vi "ControlEnhanced - BackupCopy.vi"() -> ()   [LabVIEW 2018]
uses:
  <vilib>/Platform/TimedLoop/XDataNode/timing_clust.ctl
  <vilib>/Platform/TimedLoop/XDataNode/nitl_modes.ctl
  <vilib>/Platform/TimedLoop/XDataNode/wakeup.ctl
  <vilib>/myRIO/Instrument Drivers/Onboard IO/AI/typedefs/AI Reference.ctl
  <vilib>/myRIO/Common/Instrument Driver Framework/Utilities/typedefs/myRIO Generic Hardware Reference.ctl
  <vilib>/myRIO/Common/Instrument Driver Framework/Utilities/typedefs/Hardware Version Enum.ctl
  <vilib>/myRIO/Common/Instrument Driver Framework/Utilities/typedefs/myRIO v1.0 Reference.ctl
  <vilib>/myRIO/Common/Instrument Driver Framework/Utilities/typedefs/Generic FPGA Reference.ctl
  <vilib>/myRIO/Common/Instrument Driver Framework/myRIO v1.0/AI/typedefs/AI Channels List.ctl
  <vilib>/myRIO/Common/Instrument Driver Framework/myRIO v1.0/AI/typedefs/AI Channels Enum.ctl
  <vilib>/myRIO/Common/Instrument Driver Framework/Utilities/typedefs/Analog Scaling Constants List.ctl
  <vilib>/myRIO/Common/Instrument Driver Framework/Utilities/typedefs/Analog Scaling Constants.ctl
  <vilib>/userdefined/High Color/nirio_resource_hc.ctl
  <vilib>/myRIO/Instrument Drivers/Onboard IO/AO/typedefs/AO Reference.ctl
  <vilib>/myRIO/Common/Instrument Driver Framework/myRIO v1.0/AO/typedefs/AO Channels List.ctl
  <vilib>/myRIO/Common/Instrument Driver Framework/myRIO v1.0/AO/typedefs/AO Channels Enum.ctl
  <vilib>/myRIO/Common/Instrument Driver Framework/Utilities/vis/Is FPGA Ref Available.vi
  <vilib>/myRIO/Common/Instrument Driver Framework/myRIO v1.0/AI/vis/myRIO v1.1 Open AI.vi
  <vilib>/myRIO/Instrument Drivers/Onboard IO/AI/vis/Read.vi
  <vilib>/myRIO/Common/Instrument Driver Framework/myRIO v1.0/AO/vis/myRIO v1.1 Open AO.vi
  <vilib>/myRIO/Instrument Drivers/Onboard IO/AO/vis/Write.vi
  <vilib>/myRIO/Common/Instrument Driver Framework/Utilities/vis/Validate Channels.vi
  <vilib>/myRIO/Common/Instrument Driver Framework/myRIO v1.0/AI/vis/myRIO v1.0 Reserve AI.vi
  <vilib>/myRIO/Common/Instrument Driver Framework/myRIO v1.0/AO/vis/myRIO v1.0 Reserve AO.vi
  <vilib>/myRIO/Common/Instrument Driver Framework/myRIO v1.0/AI/vis/myRIO v1.0 Build MUX Configuration AI.vi
  <vilib>/myRIO/Common/Instrument Driver Framework/myRIO v1.0/Resource Manager/vis/myRIO v1.0 Reserve Channel List.vi
  <vilib>/myRIO/Common/Instrument Driver Framework/myRIO v1.0/AO/vis/myRIO v1.0 Build MUX Configuration AO.vi
  <vilib>/myRIO/Common/Instrument Driver Framework/myRIO v1.0/Resource Manager/vis/myRIO v1.0 Reserve Channel.vi
  <vilib>/myRIO/Common/Instrument Driver Framework/myRIO v1.0/Resource Manager/vis/myRIO v1.0 Unreserve Channel.vi
  <vilib>/myRIO/Common/Instrument Driver Framework/myRIO v1.0/Resource Manager/vis/myRIO v1.0 Build Mutex Name.vi
  <vilib>/Utility/VariantDataType/GetNumericInfo.vi
  <vilib>/Utility/error.llb/Error Cluster From Error Code.vi
  <vilib>/myRIO/Common/Instrument Driver Framework/myRIO v1.0/myRIO v1.1 Open.vi
  <vilib>/myRIO/Common/Instrument Driver Framework/myRIO v1.0/AI/vis/myRIO v1.0 Get Scaling Constants AI.vi
  <vilib>/myRIO/Common/Instrument Driver Framework/Utilities/vis/IO Manager.vi
  <vilib>/myRIO/Common/Instrument Driver Framework/Utilities/vis/Configuration Manager.vi
  <vilib>/myRIO/Common/Instrument Driver Framework/myRIO v1.0/myRIO v1.0 Close.vi
  <vilib>/myRIO/Common/Instrument Driver Framework/myRIO v1.0/AI/vis/myRIO v1.0 Read AI.vi
  <vilib>/myRIO/Common/Instrument Driver Framework/myRIO v1.0/AO/vis/myRIO v1.0 Get Scaling Constants AO.vi
  <vilib>/myRIO/Common/Instrument Driver Framework/myRIO v1.0/AO/vis/myRIO v1.0 Write AO.vi
  <vilib>/platform/TimedLoop/XDataNode/XDataNode.xnode
  <vilib>/myRIO/Express VI/Onboard IO/AI/AI Express VI.xnode
  <vilib>/myRIO/Instrument Drivers/Onboard IO/AI/vis/myRIO AI Open.xnode
  <vilib>/myRIO/Express VI/Onboard IO/AO/AO Express VI.xnode
  <vilib>/myRIO/Instrument Drivers/Onboard IO/AO/vis/myRIO AO Open.xnode
  <vilib>/myRIO/Instrument Drivers/Onboard IO/AI/AI.lvlib
  <vilib>/myRIO/Instrument Drivers/Onboard IO/AO/AO.lvlib
  <vilib>/Platform/TimedLoop/XDataNode/XDNodeRunTimeDep.lvlib
panel:
  in  "Blank Button 3":bool caption="Blank Button"
  in  "Blank Button":bool
  in  "Blank Button 2":bool caption="Blank Button"
  in  "Blank Button":bool
  in  "SoVal":bool
  in  "Gas Reg\n(Manual)":dbl
  in  "OK Button":bool
  in  "SELF-DESTRUCT BUTTON":bool
  in  "Operating Mode":string(combo)="1"
  in  "Upper \nBound":dbl=0.1 format="%#_13g"
  in  "Lower \nBound":dbl=0.04 format="%#_13g"
  in  "Signal Frequency / Hz":i64=200
  in  "Factor of Decrease":dbl=1e-05
  in  "Factor of Increase":dbl=1e-05
  out "SoVal":bool
  in  "BIGGER SELF-DESTRUCT BUTTON":bool
  out "SoVal\nSoVal (C/AO0 (AO0))":dbl
  out "Gas Reg. (A/AO0 (Pin 2))":dbl=0.04 min=0.04 max=0.1
  in  "Setpoint":dbl=5.5
  out "Force Resistor":dbl
  out "FSR Dial":dbl(knob) scale=-9.0..11.0
  out "PP 2":dbl
  out "PP Dial":dbl(knob) scale=-11.0..11.0
  out "PP":bool
  out "FSR":bool
  in  "PP Weight":dbl=0.1 min=0.0 max=1.0 step=0.001
  in  "FSR Weight":dbl=0.1 min=0.0 max=1.0 step=0.0001
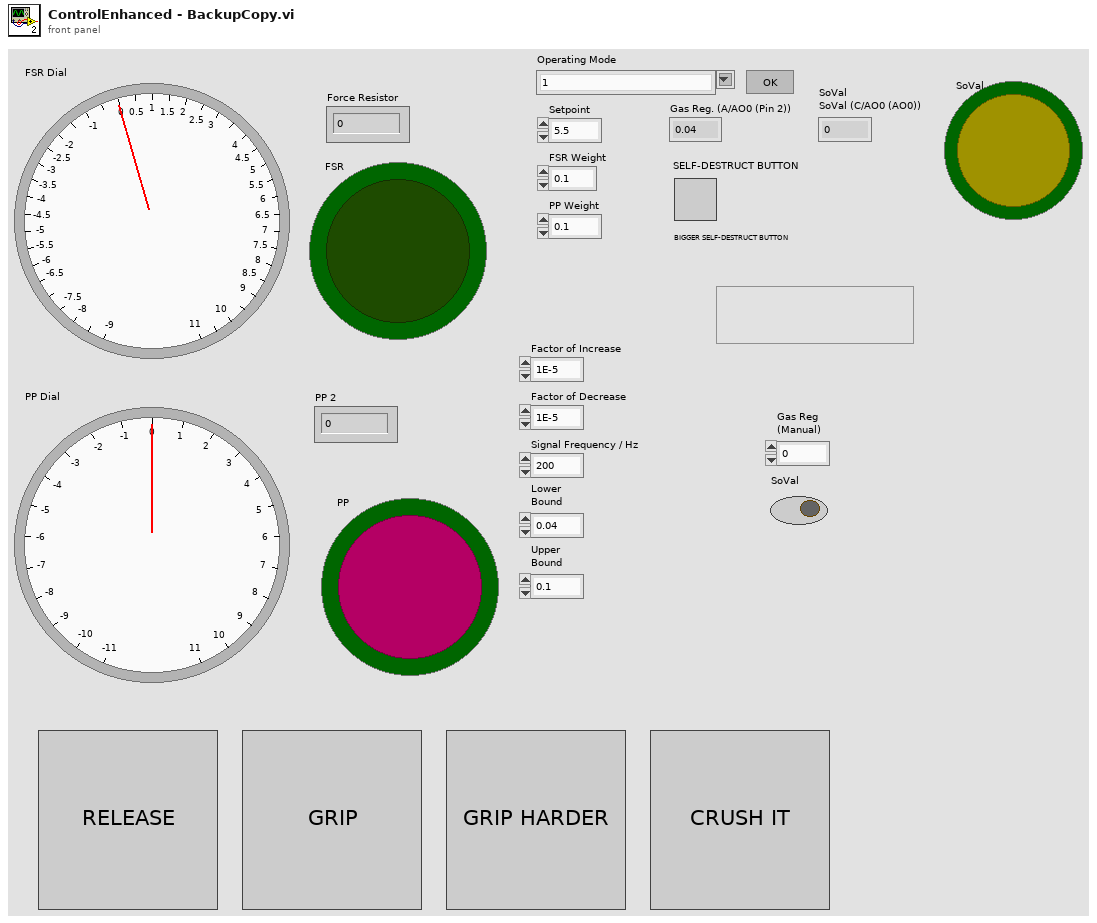
[diagram p1: front panel]
types:
  T1 = typedef "XDNodeRunTimeDep.lvlib/timing_clust.ctl" = cluster{"Expected End [f-1]":u64, "Actual End [f-1]":u64, "Finished Late? [f-1]":bool, "Expected End [i-1]":u64, "Actual End [i-1]":u64, "Finished Late? [i-1]":bool, "Expected Start [i]":u64, "Actual Start [i]":u64, "Expected Start [f]":u64, "Actual Start [f]":u64, "Source Name":string, "Structure Name":string, "Period":i64, "Deadline":i64, "Offset":i64, "Start":i64, "Priority":i32, "Timeout":i32, "Mode":T2, "Wakeup Reason":T3, "Error":errorcluster, "Source Type":string, "Secondary Source Type":string, "Global End Time":u64, "Global Start Time":u64, "Frame Duration":u64, "Iteration Duration":u64, "Assigned CPU":i32, "I/O Scan Engine Mode":u32}
  T2 = typedef "XDNodeRunTimeDep.lvlib/nitl_modes.ctl" = enum32{"No Change", "Process missed periods, maintain original phase", "Discard missed periods, maintain original phase", "Process missed periods, ignore original phase", "Discard missed periods, ignore original phase"}
  T3 = typedef "XDNodeRunTimeDep.lvlib/wakeup.ctl" = enum32{"Normal", "Aborted", "Asynchronous wakeup", "Timing source error", "Timed loop error", "Timeout"}
  T4 = typedef "AO.lvlib/AO Reference.ctl" = cluster{"myRIO Reference":T5, "AO Channel List":T9, "AO Scaling Constant List":T11}
  T5 = typedef "myRIO Generic Hardware Reference.ctl" = cluster{"myRIO Model":T6, "myRIO Hardware Reference":T7}
  T6 = typedef "Hardware Version Enum.ctl" = enum16{"Unknown", "myRIO-1900", "myRIO-1950", "roboRIO", "NI ELVIS RIO CM", "ELVIS III"}
  T7 = typedef "myRIO v1.0 Reference.ctl" = cluster{"Generic FPGA Reference":T8, "Allow multiple opens":bool}
  T8 = typedef "Generic FPGA Reference.ctl" = refnum<k20>
  T9 = typedef "AO Channels List.ctl" = T10[]
  T10 = typedef "AO Channels Enum.ctl" = enum16{"Not Connected", "AudioOut/Left", "AudioOut/Right", "C/AO0", "C/AO1", "A/AO0", "A/AO1", "B/AO0", "B/AO1"}
  T11 = typedef "Analog Scaling Constants List.ctl" = T12[]
  T12 = typedef "Analog Scaling Constants.ctl" = cluster{"LSB Weight (Volts)":dbl, "Offset (Volts)":dbl, "Signed?":bool}
  T13 = typedef "nirio_resource_hc.ctl" = tag
  T14 = typedef "AI.lvlib/AI Reference.ctl" = cluster{"myRIO Reference":T5, "AI Channels List":T15, "AI Scaling Constants List":T11}
  T15 = typedef "AI Channels List.ctl" = T16[]
  T16 = typedef "AI Channels Enum.ctl" = enum16{"Not Connected", "AudioIn/Left", "AudioIn/Right", "C/AI0", "C/AI1", "A/AI0", "A/AI1", "A/AI2", "A/AI3", "A/AI4", "A/AI5", "A/AI6", "A/AI7", "B/AI0", "B/AI1", "B/AI2", "B/AI3", "B/AI4", "B/AI5", "B/AI6", "B/AI7", "AI/AI0", "AI/AI1", "AI/AI2", "AI/AI3", "A/AI0 (DIFF)", "A/AI1 (DIFF)", "A/AI2 (DIFF)", "A/AI3 (DIFF)", "B/AI0 (DIFF)", "B/AI1 (DIFF)", "B/AI2 (DIFF)", "B/AI3 (DIFF)"}
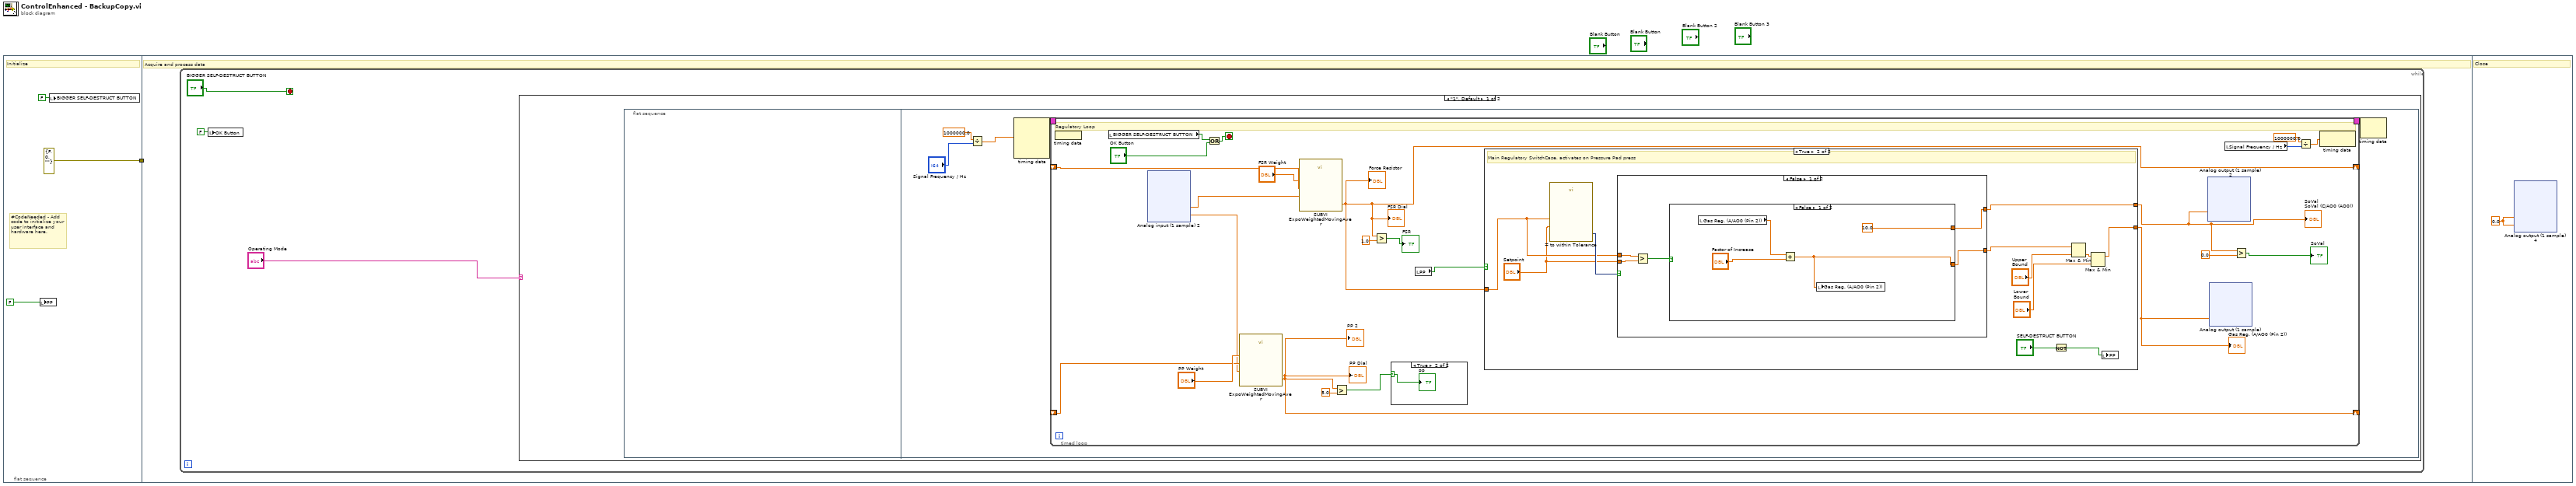
[diagram p0: block diagram]
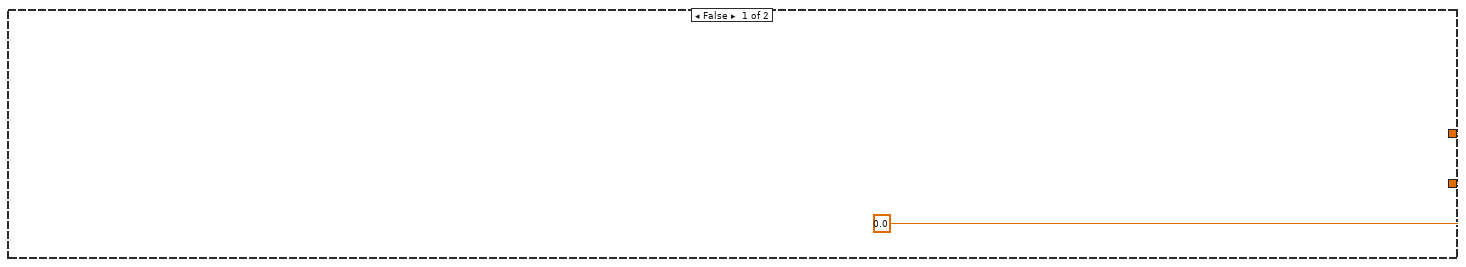
[diagram p2: hidden frame]
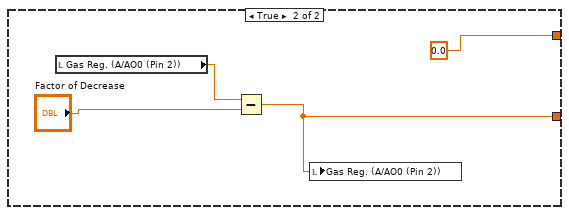
[diagram p3: hidden frame]
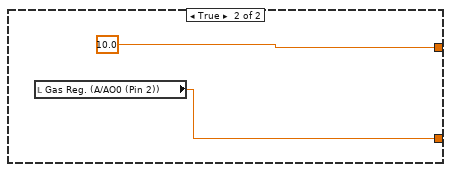
[diagram p4: hidden frame]
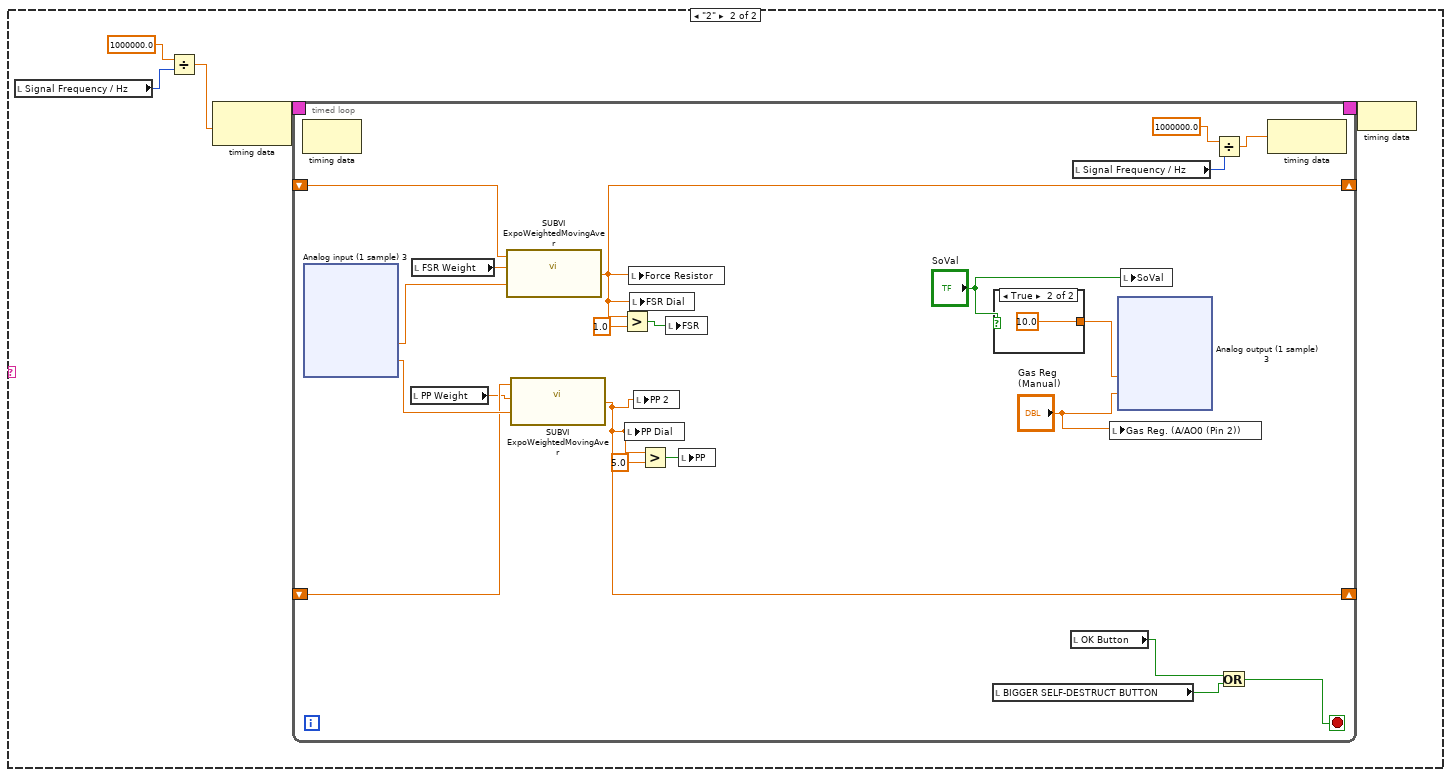
[diagram p6: hidden frame]
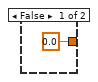
[diagram p7: hidden frame]
diagram:
  n1 = flat-sequence {
    tunnel: [errorcluster {"status"=FALSE, "code"=0, "source"=""} ("error in (no error)")] -> w1
    tunnel: w1 -> [_]
    frame #0 {
      # "#CodeNeeded - Add code to initialize your user interface and hardware here."
      # "Initialize"
      n2 = local write "PP"(FALSE ("PP")) -> ()
      n3 = local write "BIGGER SELF-DESTRUCT BUTTON"(FALSE ("BIGGER SELF-DESTRUCT BUTTON")) -> ()
    }
    frame #1 {
      # "Acquire and process data"
      n4 = while {
        stop <- "BIGGER SELF-DESTRUCT BUTTON" stop-if-true
        n5 = local write "OK Button"(FALSE ("OK Button")) -> ()
        n6 = case shown="\"1\", Default" "Operating Mode" {
          frame "1", Default {
            n7 = flat-sequence {
              frame #0 {
              }
              frame #1 {
                n8 = Divide(x=1000000.0, y="Signal Frequency / Hz") -> (x/y=w10:dbl)
                n9 = node-c288(w10) -> (w12:T1)  [unwired: 3 in]
                n10 = timed-loop "Timed Loop" {
                  shift-right: [w30] -> _
                  shift-left: _ -> [w31]
                  shift-right: [w24] -> _
                  shift-left: _ -> [w28]
                  timing: w12 -> [_]
                  timing-out: [_] -> w11
                  stop <- w16 stop-if-true
                  # "Regulatory Loop"
                  n11 = node-c288() -> ()  [unwired: 1 in]
                  n12 = local read "BIGGER SELF-DESTRUCT BUTTON"() -> (w17:bool)
                  n13 = xnode "Analog input (1 sample) 2"() -> ("FSR (C/AI0 (AI0))"=w29:dbl, "PressurePad (C/AI1 (AI1))"=w14:dbl)  [unwired: 1 in, 1 out]
                  n14 = Or(x=w17, y="OK Button") -> (x .or. y?=w16:bool)
                  n15 = call "SUBVI ExpoWeightedMovingAver.vi"("New Sample"=w14, "EWMA Weight"="PP Weight", "Old Estimate"=w31) -> ("Weighted Average"=w30:dbl)  [unwired: 8 in]
                  "PP 2" <- w30
                  "PP Dial" <- w30
                  n16 = call "SUBVI ExpoWeightedMovingAver.vi"("New Sample"=w29, "EWMA Weight"="FSR Weight", "Old Estimate"=w28) -> ("Weighted Average"=w24:dbl)  [unwired: 8 in]
                  "Force Resistor" <- w24
                  "FSR Dial" <- w24
                  n17 = Greater?(x=w30, y=5.0) -> (0:w26:bool)
                  n18 = Greater?(x=w24, y=1.0) -> (0:→"FSR":bool)
                  n19 = case shown="True" w26 {
                    selector: w26 -> [_ w141]
                    frame False {
                    }
                    frame True {
                      "PP" <- w141
                    }
                  }
                  n20 = local read "PP"() -> (w25:bool)
                  n21 = case shown="True" w25 {
                    tunnel: w24 -> [_ w124]
                    tunnel: [w114 w117] -> w23
                    tunnel: [w114 w120] -> w13
                    frame False {
                      w114 = 0.0
                    }
                    frame True {
                      # "Main Regulatory SwitchCase, activates on Pressure Pad press"
                      n22 = call "= to within Tolerance"("Constant Value to Compare Against"="Setpoint", "Operand 1"=w124) -> ("Result"=w125:dynamicdata)  [unwired: 8 in, 1 out]
                      n23 = case shown="False" w125 {
                        tunnel: [w127 w140] -> w122
                        tunnel: w124 -> [w130 _]
                        tunnel: "Setpoint" -> [w129 _]
                        tunnel: [w126 10.0 ("SoVal\nSoVal (C/AO0 (AO0))")] -> w120
                        frame False {
                          n24 = Greater?(x=w130, y=w129) -> (0:w128:bool)
                          n25 = case shown="False" w128 {
                            tunnel: [w134 w137] -> w127
                            tunnel: [10.0 0.0] -> w126
                            frame False {
                              n26 = local read "Gas Reg. (A/AO0 (Pin 2))"() -> (w133:dbl)
                              n27 = Add(x=w133, y="Factor of Increase") -> (x+y=w134:dbl)
                              n28 = local write "Gas Reg. (A/AO0 (Pin 2))"(w134) -> ()
                            }
                            frame True {
                              n29 = local read "Gas Reg. (A/AO0 (Pin 2))"() -> (w138:dbl)
                              n30 = Subtract(x=w138, y="Factor of Decrease") -> (x-y=w137:dbl)
                              n31 = local write "Gas Reg. (A/AO0 (Pin 2))"(w137) -> ()
                            }
                          }
                        }
                        frame True {
                          n32 = local read "Gas Reg. (A/AO0 (Pin 2))"() -> (w140:dbl)
                        }
                      }
                      n33 = Not(x="SELF-DESTRUCT BUTTON") -> (.not. x?=w115:bool)
                      n34 = Max & Min(x=w122, y="Upper \nBound") -> (min(x,y)=w119:dbl)  [unwired: 1 out]
                      n35 = Max & Min(x=w119, y="Lower \nBound") -> (max(x,y)=w117:dbl)  [unwired: 1 out]
                      n36 = local write "PP"(w115) -> ()
                    }
                  }
                  "Gas Reg. (A/AO0 (Pin 2))" <- w23
                  "SoVal\nSoVal (C/AO0 (AO0))" <- w13
                  n37 = xnode "Analog output (1 sample) 2"("SoVal (C/AO0 (AO0))"=w13) -> ()  [unwired: 1 in, 1 out]
                  n38 = xnode "Analog output (1 sample)"("Gas Reg. (A/AO0 (Pin 2))"=w23) -> ()  [unwired: 1 in, 1 out]
                  n39 = local read "Signal Frequency / Hz"() -> (w19:i64)
                  n40 = Greater?(x=w13, y=0.0) -> (0:→"SoVal":bool)
                  n41 = Divide(x=1000000.0, y=w19) -> (x/y=w18:dbl)
                  n42 = node-c288(w18) -> ()  [unwired: 1 out]
                }
                n43 = node-c288(w11) -> ()  [unwired: 1 out]
              }
            }
          }
          frame "2" {
            n44 = local read "Signal Frequency / Hz"() -> (w188:i64)
            n45 = Divide(x=1000000.0, y=w188) -> (x/y=w184:dbl)
            n46 = node-c288(w184) -> (w186:T1)
            n47 = timed-loop {
              timing: w186 -> [_]
              timing-out: [_] -> w185
              shift-right: [w200] -> _
              shift-left: _ -> [w204]
              shift-right: [w197] -> _
              shift-left: _ -> [w203]
              stop <- w189 stop-if-true
              n48 = node-c288() -> ()  [unwired: 1 in, 1 out]
              n49 = xnode "Analog input (1 sample) 3"() -> ("FSR (C/AI0 (AI0))"=w206:dbl, "PressurePad (C/AI1 (AI1))"=w205:dbl)  [unwired: 1 in, 1 out]
              n50 = local read "PP Weight"() -> (w201:dbl)
              n51 = local read "FSR Weight"() -> (w202:dbl)
              n52 = call "SUBVI ExpoWeightedMovingAver.vi"("New Sample"=w206, "EWMA Weight"=w202, "Old Estimate"=w204) -> ("Weighted Average"=w200:dbl)  [unwired: 8 in]
              n53 = call "SUBVI ExpoWeightedMovingAver.vi"("New Sample"=w205, "EWMA Weight"=w201, "Old Estimate"=w203) -> ("Weighted Average"=w197:dbl)  [unwired: 8 in]
              n54 = Greater?(x=w200, y=1.0) -> (0:w199:bool)
              n55 = local write "PP Dial"(w197) -> ()
              n56 = local write "Force Resistor"(w200) -> ()
              n57 = local write "FSR Dial"(w200) -> ()
              n58 = local write "PP 2"(w197) -> ()
              n59 = Greater?(x=w197, y=5.0) -> (0:w196:bool)
              n60 = local write "FSR"(w199) -> ()
              n61 = local write "PP"(w196) -> ()
              n62 = local read "BIGGER SELF-DESTRUCT BUTTON"() -> (w190:bool)
              n63 = case shown="True" "SoVal" {
                tunnel: [0.0 10.0] -> w193
                frame False {
                }
                frame True {
                }
              }
              n64 = local read "OK Button"() -> (w191:bool)
              n65 = local read "Signal Frequency / Hz"() -> (w208:i64)
              n66 = local write "Gas Reg. (A/AO0 (Pin 2))"("Gas Reg\n(Manual)") -> ()
              n67 = xnode "Analog output (1 sample) 3"("SoVal (C/AO0 (AO0))"=w193, "Gas Reg (A/AO0 (Pin 2))"="Gas Reg\n(Manual)") -> ()  [unwired: 1 in, 1 out]
              n68 = local write "SoVal"("SoVal") -> ()
              n69 = Divide(x=1000000.0, y=w208) -> (x/y=w207:dbl)
              n70 = Or(x=w191, y=w190) -> (x .or. y?=w189:bool)
              n71 = node-c288(w207) -> ()  [unwired: 1 out]
            }
            n72 = node-c288(w185) -> ()
          }
        }
      }
    }
    frame #2 {
      w296 = 0.0
      # "Close"
      n73 = xnode "Analog output (1 sample) 4"("C/AO0 (AO0)"=w296, "A/AO0 (Pin 2)"=w296) -> ()  [unwired: 1 in, 1 out]
    }
  }
